vi "Capacitance Estimator.vi"(1 "normalized waveform":waveform(dbl)={"t0"=timestamp(3087922235.213 s since 1904-01-01), "dt"=1.9999999494757503e-05, "Y"=array[1000 elements]}, 2 "Resistance (Ohms)":dbl=100000.0 format="%.4e") -> (0 "Estimated Capacitance (F)":dbl=1.269612045289484e-08 format="%.4e")   [LabVIEW 2014]
doc: "Capacitance Estimator\n\nGiven an RC decay waveform and the resistance R(ohms), this vi estimates the Capacitance (F).\n\nTau = Fractional index at 1/e * dt \nCapacitance = Tau / resistance\n\nBeverly Abadines\nPHY 350\nP6"
panel:
  # "C(T) Capacitance Estimator"
  # "Beverly Abadines\nPHY 350\nP6"
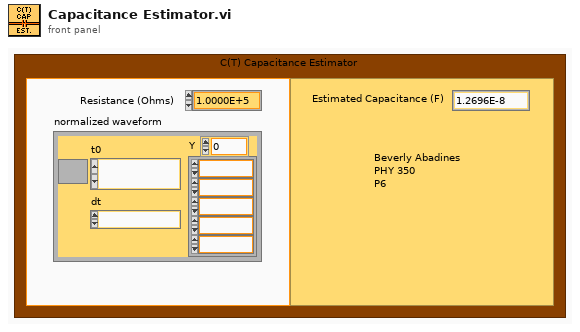
[diagram p1: front panel]
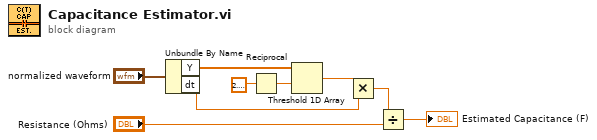
[diagram p0: block diagram]
diagram:
  n1 = Unbundle By Name("normalized waveform") -> ("Y"=w7:dbl[], "dt"=w3:dbl)
  n2 = Reciprocal(x=2.718281828459045) -> (1/x=w5:dbl)
  n3 = Threshold 1D Array(2:w5, 3:w7) -> (0:w4:dbl)  [unwired: 1 out]
  n4 = Multiply(x=w4, y=w3) -> (x*y=w2:dbl)
  n5 = Divide(x=w2, y="Resistance (Ohms)") -> (x/y=→"Estimated Capacitance (F)":dbl)
